vi "Method_Const.vi"(4 "Value":timestamp, 5 "Input A":refnum<class "Abs_Time.lvclass">) -> (1 "Result":refnum<class "Abs_Double Float.lvclass">)   [LabVIEW 2021, in "Subtract_Time-Time.lvclass"]
uses:
  Subtract_Time-Time.lvclass
  Abs_Types/Time/Abs_Time.lvclass
  Abs_Types/Double Float/Abs_Double Float.lvclass
  C:/Program Files (x86)/National Instruments/LabVIEW 2021/vi.lib/TSA/Abstract Data Classes/Abs_Types/Double Float/Abs_Double Float.lvclass
  Subtract_Time-Time.lvclass/Subtract_Time-Time.ctl
  Properties/Write Input A.vi
  Properties/Write Input B.vi
  Constants/Support/Time/Const_Time.lvclass
  C:/Program Files (x86)/National Instruments/LabVIEW 2021/vi.lib/TSA/Abstract Data Classes/Abs_Types/Time/Abs_Time.lvclass
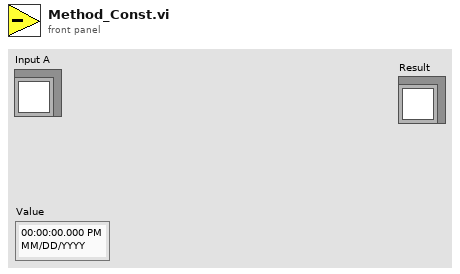
[diagram p1: front panel]
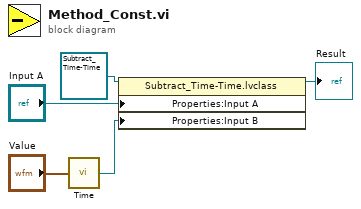
[diagram p0: block diagram]
diagram:
  n1 = call "Time.vi"("Value"="Value") -> ("Constant"=w2:refnum<class "Const_Time.lvclass">)  [unwired: 4 in]
  n2 = property class="Subtract_Time-Time.lvclass"(reference=refnum<class "Subtract_Time-Time.lvclass"> refnum ("Subtract_DBL.lvclass"), "Properties:Input A"="Input A", "Properties:Input B"=w2) -> (reference out=→"Result":refnum<class "Subtract_Time-Time.lvclass">)  [unwired: 1 in, 1 out]
